vi "Write On.vi"(8 "error in (no error)":errorcluster, 10 "On":bool, 11 "ControlHumidifierPump in":refnum<class "ControlHumidifierPump.lvclass">) -> (0 "error out":errorcluster, 3 "ControlHumidifierPump out":refnum<class "ControlHumidifierPump.lvclass">)   [LabVIEW 2014, in "Controller.lvlib" / "ControlHumidifierPump.lvclass"]
uses:
  ControlHumidifierPump.lvclass
  ControlHumidifierPump.lvclass/ControlHumidifierPump.ctl
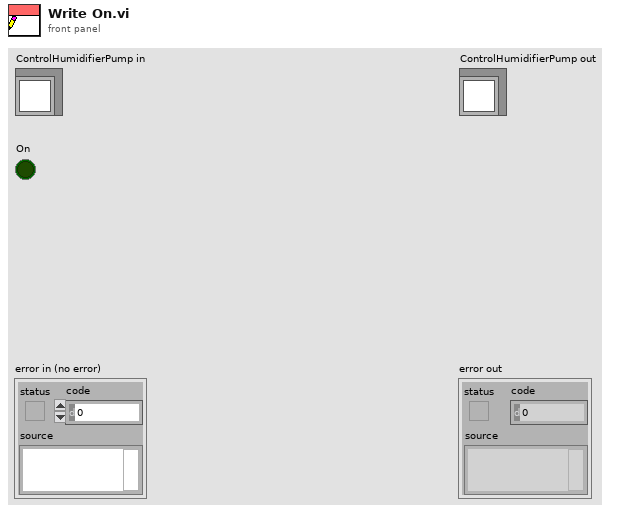
[diagram p1: front panel]
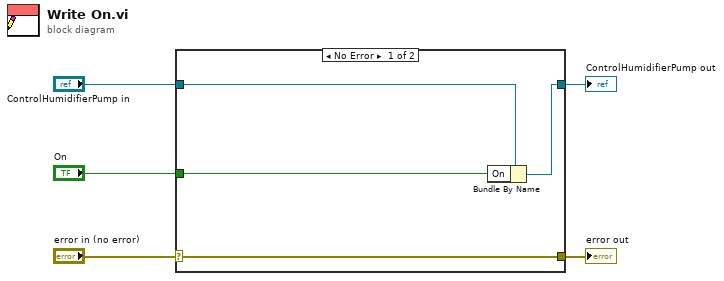
[diagram p0: block diagram]
diagram:
  n1 = case shown="No Error" "error in (no error)" {
    selector: "error in (no error)" -> [w9 w10]
    tunnel: [w9 w10] -> w4
    tunnel: [w7 w11] -> w2
    tunnel: "ControlHumidifierPump in" -> [w8 w11]
    tunnel: "On" -> [w6 _]
    frame No Error {
      n2 = Bundle By Name(cluster=w8, "On"=w6) -> (w7:refnum<class "ControlHumidifierPump.lvclass">)
    }
    frame Error {
    }
  }
  "error out" <- w4
  "ControlHumidifierPump out" <- w2
